vi "Display Console Main.vi"(8 "error in (no error)":errorcluster) -> (0 "error out":errorcluster)   [LabVIEW 2020, in "Display Console.lvlib"]
doc: "This is the Main VI for the Display Console Module."
uses:
  Display Console.lvlib
  Private Controls/FG Actions.ctl
  Private Controls/Message enum.ctl
  Private Controls/Message Cluster.ctl
  Private Controls/Module Data.ctl
panel:
  out "Transaction":string
  out "Message Screen":string
  out "Card Read":bool
  # "[Covers: UI1]"
  # "[Covers: UI3]"
  # "[Covers: UI3A"
  # "[Covers: UI3B]"
  # "[Covers: UI3C]"
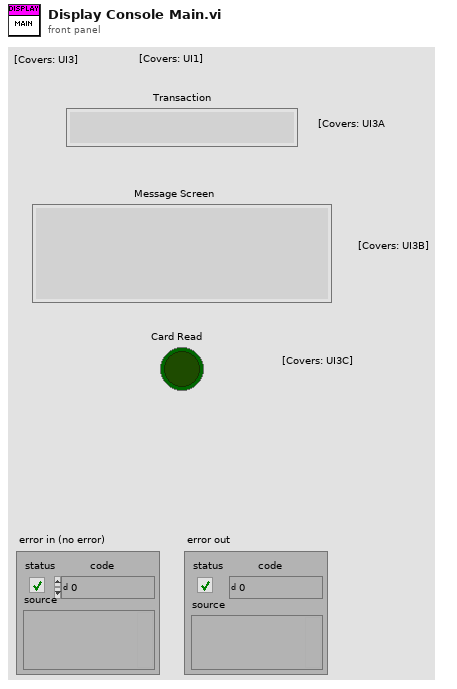
[diagram p1: front panel]
types:
  T1 = typedef "Display Console.lvlib/Module Data.ctl" = cluster{"Card Read":bool, "Message Screen":string, "Transaction":string}
  T2 = typedef "Display Console.lvlib/FG Actions.ctl" = enum16{"Get", "Set", "Clear"}
  T3 = typedef "Display Console.lvlib/Message Cluster.ctl" = cluster{"Message":T4, "Data":variant}
  T4 = typedef "Display Console.lvlib/Message enum.ctl" = enum16{"Initialize", "Update Message", "Terminate State", "Error", "Exit"}
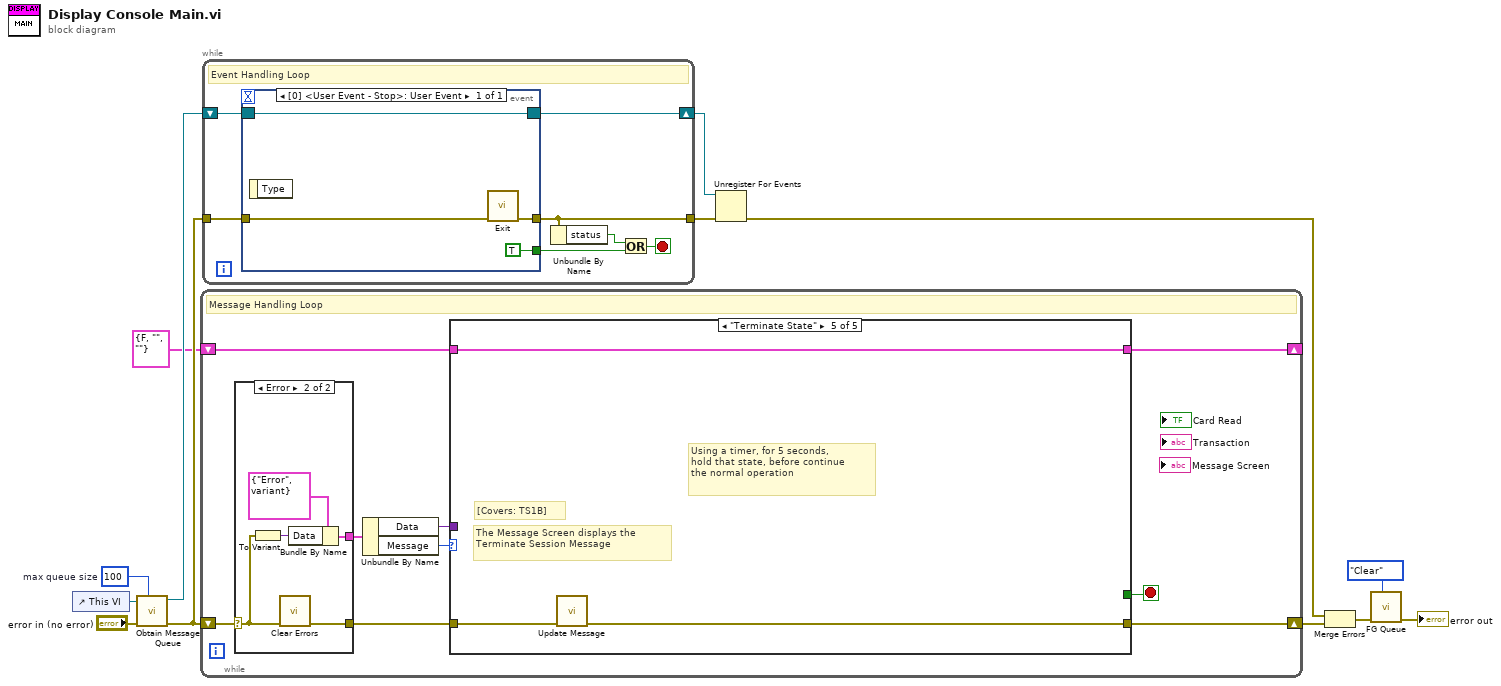
[diagram p0: block diagram]
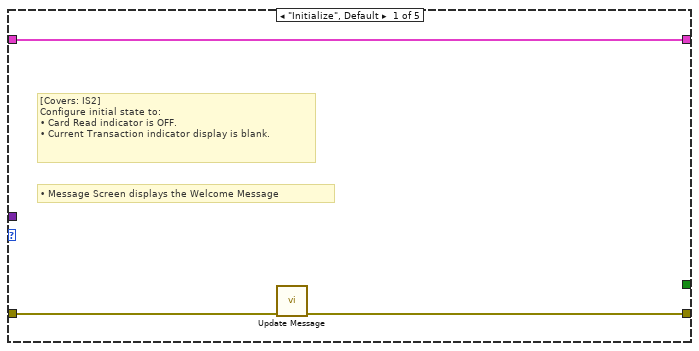
[diagram p2: hidden frame]
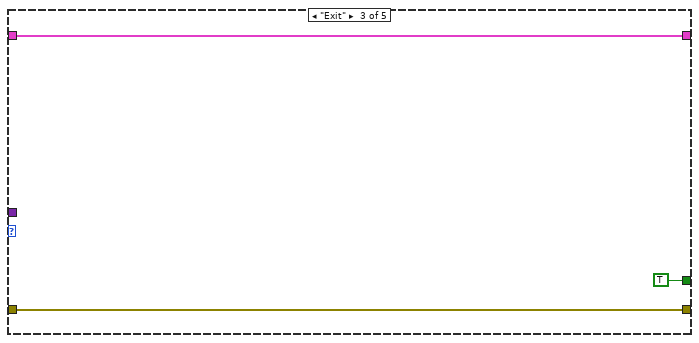
[diagram p4: hidden frame]
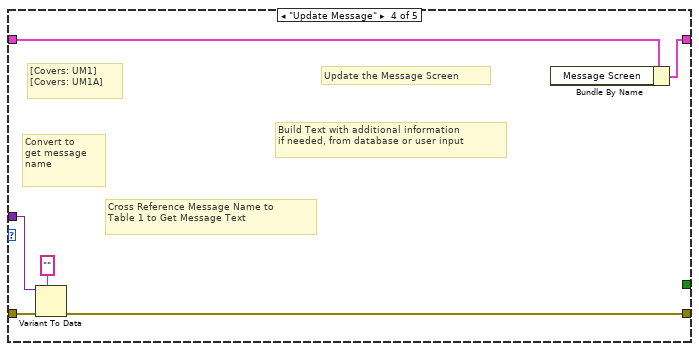
[diagram p5: hidden frame]
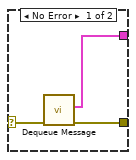
[diagram p6: hidden frame]
diagram:
  w7 = 100  # max queue size
  n1 = control-ref of="This VI"() -> (w8:refnum<vi>)
  n2 = call "Obtain Message Queue.vi"("max queue size (-1, unlimited)"=w7, "error in (no error)"="error in (no error)", "VI Reference"=w8) -> ("error out"=w3:errorcluster, "Event Registration Refnum"=w10:refnum<event-registration>)  [unwired: 7 in]
  n3 = while {
    shift-right: [w17] -> w13
    shift-left: w3 -> [w22]
    shift-right: [w14] -> _
    shift-left: T1 {"Card Read"=FALSE, "Message Screen"="", "Transaction"=""} ("Message Cluster") -> [w15]
    stop <- w16 stop-if-true
    # "Message Handling Loop"
    n4 = case shown="Error" w22 {
      selector: w22 -> [w40 w46]
      tunnel: [w41 w47] -> w18
      tunnel: [w42 w43] -> w21
      frame No Error {
        n5 = call "Dequeue Message.vi"("error in (no error)"=w40) -> ("error out"=w41:errorcluster, "Element"=w42:T3)  [unwired: 9 in]
      }
      frame Error {
        n6 = To Variant(anything=w46) -> (Variant=w44:variant)
        n7 = call <vilib>:"Clear Errors.vi"("error in (no error)"=w46) -> ("error out"=w47:errorcluster)  [unwired: 5 in, 1 out]
        n8 = Bundle By Name(cluster=T3 {"Message"=enum."Error", "Data"=variant} ("Message Cluster"), "Data"=w44) -> (w43:T3)
      }
    }
    n9 = Unbundle By Name(w21) -> ("Data"=w19:variant, "Message"=w20:T4)
    n10 = case shown="\"Terminate State\"" w20 {
      tunnel: w19 -> [_ _ _ w35 _]
      tunnel: w18 -> [w24 w27 w30 w34 w38]
      tunnel: [w23 w27 w30 w33 w37] -> w17
      tunnel: [_ _ TRUE _ _] -> w16
      tunnel: w15 -> [w25 w26 w28 w32 w39]
      tunnel: [w25 w26 w28 w31 w39] -> w14
      frame "Initialize", Default {
        # "• Message Screen displays the Welcome Message"
        # "[Covers: IS2]\nConfigure initial state to:\n• Card Read indicator is OFF.\n• Current Transaction indicator display is blank."
        n11 = call "Update Message.vi"("error in (no error)"=w24) -> ("error out"=w23:errorcluster)  [unwired: 10 in]
      }
      frame "Error" {
      }
      frame "Exit" {
      }
      frame "Update Message" {
        # "[Covers: UM1] \n[Covers: UM1A]"
        # "Update the Message Screen"
        # "Build Text with additional information\nif needed, from database or user input"
        # "Cross Reference Message Name to\nTable 1 to Get Message Text"
        # "Convert to \nget message \nname"
        n12 = Variant To Data(error in=w34, type="", Variant=w35) -> (error out=w33:errorcluster)  [unwired: 1 out]
        n13 = Bundle By Name(cluster=w32) -> (w31:T1)  [unwired: 1 in]
      }
      frame "Terminate State" {
        # "Using a timer, for 5 seconds,\nhold that state, before continue\nthe normal operation"
        # "The Message Screen displays the\nTerminate Session Message"
        # "[Covers: TS1B]"
        n14 = call "Update Message.vi"("error in (no error)"=w38) -> ("error out"=w37:errorcluster)  [unwired: 10 in]
      }
    }
  }
  n15 = while {
    shift-right: [w53] -> w11
    shift-left: w10 -> [w54]
    tunnel: w3 -> [w51]
    tunnel: [w49] -> w2
    stop <- w50 stop-if-true
    # "Event Handling Loop"
    n16 = event shown="[0] <User Event - Stop>: User Event" {
      selector: w54 -> [w55]
      dyn-events: [w55] -> w53
      timeout: _ -> [_]
      tunnel: [TRUE ("Discard?")] -> w52
      tunnel: w51 -> [w57]
      tunnel: [w56] -> w49
      event User Event {
        n17 = event-data() -> ()  [unwired: 1 in, 1 out]
        n18 = call "Exit.vi"("error in (no error)"=w57) -> ("error out"=w56:errorcluster)  [unwired: 10 in]
      }
    }
    n19 = Unbundle By Name(w49) -> ("status"=w48:bool)
    n20 = Or(x=w48, y=w52) -> (x .or. y?=w50:bool)
  }
  n21 = Unregister For Events(event registration refnum=w11, error in=w2) -> (error out=w12:errorcluster)
  n22 = Merge Errors(w12, w13) -> (w5:errorcluster)
  n23 = call "FG Queue.vi"("FG Actions"=FG_Actions."Clear", "error in (no error)"=w5) -> ("error out"=→"error out":errorcluster)  [unwired: 8 in, 1 out]
